vi "Set Start Trigger (In Range).vi"(5 "Retriggerable (F)":bool, 7 "Pre-Trigger Duration (0 s)":dbl, 8 "error in (no error)":errorcluster, 9 "Trigger Channel":string, 10 "Range Options":T1, 11 "Data Logging Specification Ref in":T2) -> (0 "error out":errorcluster, 3 "Data Logging Specification Ref out":T2)   [LabVIEW 2020, in "NI_VS Data Logging API.lvlib"]
doc: "Specifies a trigger condition on which to start logging data. You also can specify whether to log channel data immediately preceding the trigger condition and whether logging is retriggerable, meaning the data logging session watches for subsequent occurrences of the start trigger after the first logging operation finishes. By default, logging stops after one operation.\n\nYou must manually select the polymorphic instance to use."
uses:
  <vilib>/NI VeriStand/Execution/DataLogging/NI_VS Data Logging API.lvlib
  <vilib>/NI VeriStand/Execution/DataLogging/DataLoggingSpecification Ref.ctl
  NationalInstruments.VeriStand.ClientAPI
  <vilib>/NI VeriStand/Execution/DataLogging/Range Options.ctl
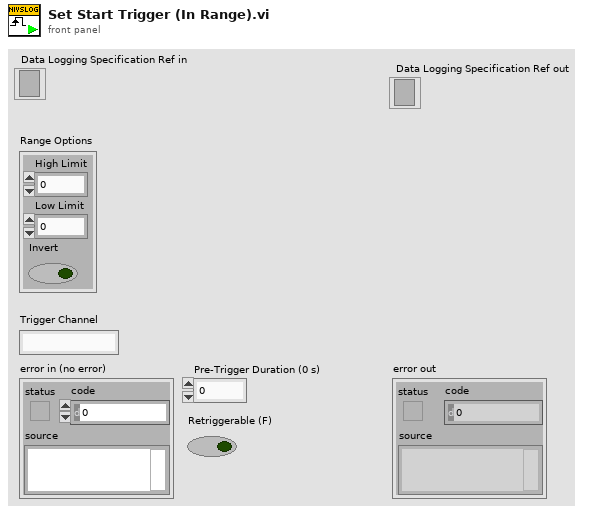
[diagram p1: front panel]
types:
  T1 = typedef "NI_VS Data Logging API.lvlib/Range Options.ctl" = cluster{"High Limit":dbl, "Low Limit":dbl, "Invert":bool}
  T2 = typedef "NI_VS Data Logging API.lvlib/DataLoggingSpecification Ref.ctl" = refnum<k24>
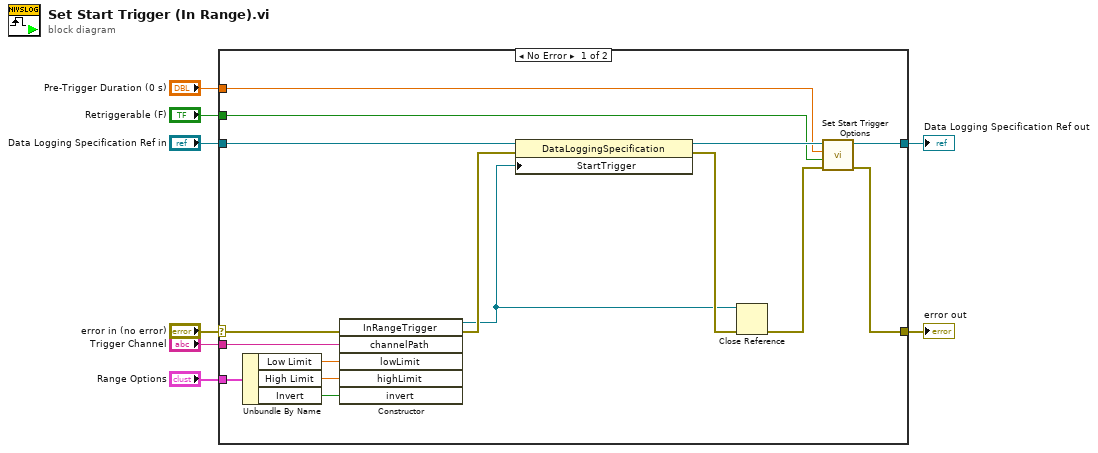
[diagram p0: block diagram]
diagram:
  n1 = case shown="No Error" "error in (no error)" {
    selector: "error in (no error)" -> [w15 w26]
    tunnel: "Data Logging Specification Ref in" -> [w23 w25]
    tunnel: [w20 w25] -> w7
    tunnel: [w19 w26] -> w6
    tunnel: "Range Options" -> [w11 _]
    tunnel: "Trigger Channel" -> [w12 _]
    tunnel: "Pre-Trigger Duration (0 s)" -> [w10 _]
    tunnel: "Retriggerable (F)" -> [w9 _]
    frame No Error {
      n2 = Unbundle By Name(w11) -> ("Low Limit"=w18:dbl, "High Limit"=w17:dbl, "Invert"=w16:bool)
      n3 = constructor class="InRangeTrigger"(error in=w15, "channelPath"=w12, "lowLimit"=w18, "highLimit"=w17, "invert"=w16) -> (reference out=w13:refnum<k24>, error out=w14:errorcluster)  [unwired: 2 in, 5 out]
      n4 = property class="DataLoggingSpecification"(reference=w23, error in=w14, "StartTrigger"=w13) -> (reference out=w22:T2, error out=w24:errorcluster)
      n5 = Close Reference(reference=w13, error in (no error)=w24) -> (error out=w21:errorcluster)
      n6 = call <vilib>:"Set Start Trigger Options.vi"("error in (no error)"=w21, "Retriggerable"=w9, "Pre-Trigger Duration"=w10, "Data Logging Specification Ref in"=w22) -> ("error out"=w19:errorcluster, "Data Logging Specification Ref out"=w20:T2)  [unwired: 6 in]
    }
    frame Error {
    }
  }
  "error out" <- w6
  "Data Logging Specification Ref out" <- w7
